vi "retrieveData.vi"(8 "error in (no error)":errorcluster, 11 "TemperatureSensor in":refnum<class "TemperatureSensor.lvclass">) -> (0 "error out":errorcluster, 2 "Temperature Measured":dbl[unit], 3 "TemperatureSensor out":refnum<class "TemperatureSensor.lvclass">)   [LabVIEW 2013, in "TemperatureSensor.lvlib" / "TemperatureSensor.lvclass"]
uses:
  <userlib>/Common/Devices/TemperatureSensor/TemperatureSensor/TemperatureSensor.lvclass
  <userlib>/Common/Devices/TemperatureSensor/TemperatureSensor/TemperatureSensor.lvclass/TemperatureSensor.ctl
  <userlib>/Common/SerialProtocols/SerialCommunicator/SerialCommunicator.lvclass
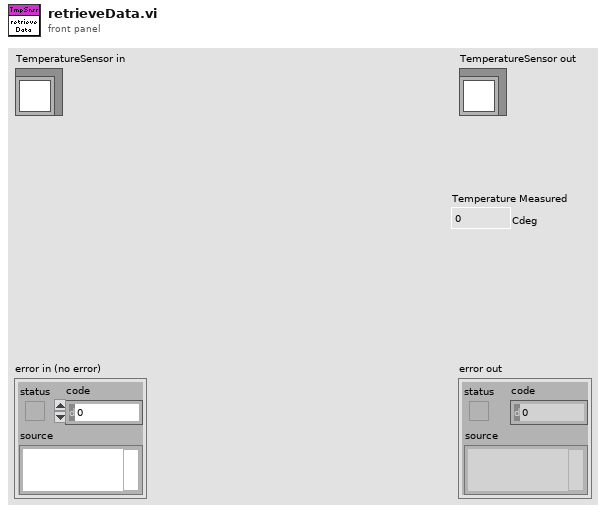
[diagram p1: front panel]
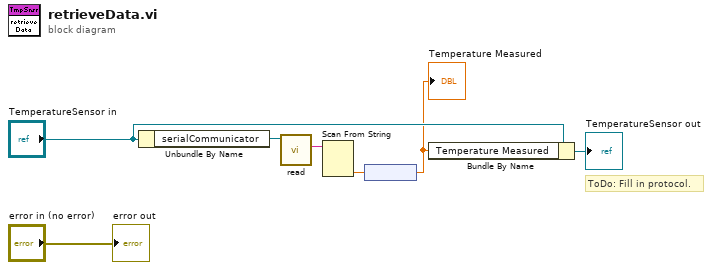
[diagram p0: block diagram]
diagram:
  # "ToDo: Fill in protocol."
  n1 = Unbundle By Name("TemperatureSensor in") -> ("serialCommunicator"=w4:refnum<class "SerialCommunicator.lvclass">)
  n2 = call-dynamic "read.vi"("SerialCommunicator in"=w4) -> ("stringRead"=w3:string)  [unwired: 8 in, 2 out]
  n3 = Scan From String(input string=w3) -> (output 1=w2:dbl)  [unwired: 4 in, 3 out]
  n4 = node(w2) -> (w1:dbl[unit])
  "Temperature Measured" <- w1
  n5 = Bundle By Name(cluster="TemperatureSensor in", "Temperature Measured"=w1) -> (→"TemperatureSensor out":refnum<class "TemperatureSensor.lvclass">)
  "error out" <- "error in (no error)"
